vi "graph coeffecient.vi"() -> ()   [LabVIEW 2009]
panel:
  out "coeffecient Array":dbl[](array[numeric])
  out "coeffecient graph":dbl[](graph)
  in  "iterations":i32
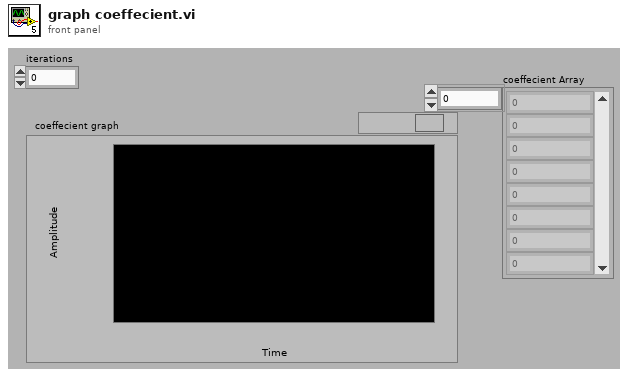
[diagram p1: front panel]
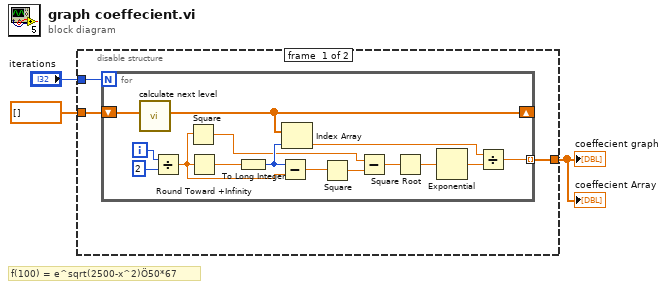
[diagram p0: block diagram]
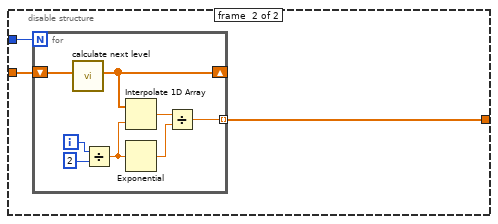
[diagram p2: hidden frame]
diagram:
  # "f(100) = e^sqrt(2500-x^2)Ö50*67"
  n1 = disable-structure shown="Enabled" {
    disable-tunnel: dbl[] [] ("next level") -> [w6 w24]
    disable-tunnel: "iterations" -> [w5 w23]
    disable-tunnel: [w4 w22] -> w1
    frame #0 {
      n2 = for {
        N: w5 -> [_]
        shift-right: [w18] -> _
        shift-left: w6 -> [w21]
        tunnel: [w12] -> w4 mode=indexing
        i -> [w20]
        n3 = call "calculate next level.vi"("pascal's triangle"=w21) -> ("next level"=w18:dbl[])  [unwired: 10 in]
        n4 = Divide(x=w20, y=2) -> (x/y=w8:dbl)
        n5 = Square(x=w8) -> (x^2=w7:dbl)
        n6 = Round Toward +Infinity(x=w8) -> (ceil(x): smallest int >= x=w11:dbl)
        n7 = To Long Integer(number=w11) -> (32bit integer=w10:i32)
        n8 = Subtract(x=w10, y=w8) -> (x-y=w9:dbl)
        n9 = Index Array(array=w18, index=w10) -> (element=w14:dbl)
        n10 = Square(x=w9) -> (x^2=w17:dbl)
        n11 = Subtract(x=w7, y=w17) -> (x-y=w16:dbl)
        n12 = Square Root(x=w16) -> (sqrt(x)=w15:dbl)
        n13 = Exponential(1:w15) -> (0:w13:dbl)
        n14 = Divide(x=w14, y=w13) -> (x/y=w12:dbl)
      }
    }
    frame #1 {
      n15 = for {
        N: w23 -> [_]
        shift-right: [w29] -> _
        shift-left: w24 -> [w32]
        tunnel: [w26] -> w22 mode=indexing
        i -> [w31]
        n16 = call "calculate next level.vi"("pascal's triangle"=w32) -> ("next level"=w29:dbl[])  [unwired: 10 in]
        n17 = Divide(x=w31, y=2) -> (x/y=w25:dbl)
        n18 = Interpolate 1D Array(1:w25, 2:w29) -> (0:w28:dbl)
        n19 = Exponential(1:w25) -> (0:w27:dbl)
        n20 = Divide(x=w28, y=w27) -> (x/y=w26:dbl)
      }
    }
  }
  "coeffecient graph" <- w1
  "coeffecient Array" <- w1
